vi "regTcpServerUserEvent.vi"(8 "error in (no error)":errorcluster, 11 "tcpServerBase in":refnum<class "TcpServerBase.lvclass">) -> (0 "error out":errorcluster, 3 "tcpServerBase out":refnum<class "TcpServerBase.lvclass">)   [LabVIEW 2018, in "TcpServerBase.lvclass"]
doc: "Register the TcpServer user event. This will be used for TcpServerCmd and TcpServerTelemetry classes."
uses:
  TcpServerBase.lvclass
  TcpServerBase.lvclass/TcpServerBase.ctl
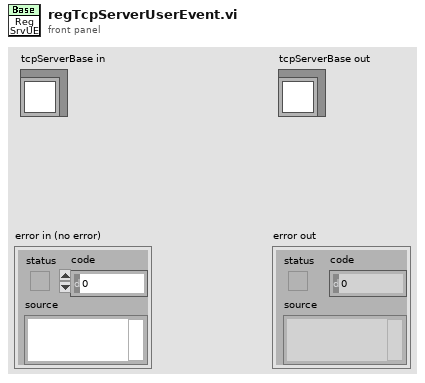
[diagram p1: front panel]
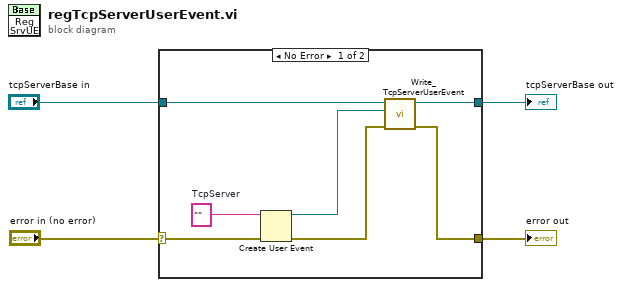
[diagram p0: block diagram]
diagram:
  n1 = case shown="No Error" "error in (no error)" {
    selector: "error in (no error)" -> [w7 w13]
    tunnel: [w9 w13] -> w3
    tunnel: [w10 w12] -> w1
    tunnel: "tcpServerBase in" -> [w11 w12]
    frame No Error {
      w8 = ""  # TcpServer
      n2 = Create User Event(user event datatype=w8, error in=w7) -> (user event=w5:refnum<user-event>, error out=w6:errorcluster)
      n3 = call "Write_TcpServerUserEvent.vi"("error in (no error)"=w6, "TcpServer"=w5, "TcpServerBase in"=w11) -> ("error out"=w9:errorcluster, "TcpServerBase out"=w10:refnum<class "TcpServerBase.lvclass">)  [unwired: 7 in]
    }
    frame Error {
    }
  }
  "error out" <- w3
  "tcpServerBase out" <- w1
